vi "Do.vi"(8 "error in (no error)":errorcluster, 10 "Actor in":refnum<class "Actor.lvclass">, 11 "Set Delays Msg":refnum<class "Set Delays Msg.lvclass">) -> (0 "error out":errorcluster, 2 "Actor out":refnum<class "Actor.lvclass">)   [LabVIEW 2021, in "BNT_DAQmx.lvlib" / "Set Delays Msg.lvclass"]
doc: "This VI delivers the message to the actor by calling the appropriate method(s) on the actor."
uses:
  Set Delays Msg.lvclass
  <vilib>/ActorFramework/Actor/Actor.lvclass
  C:/Users/Holger/Documents/LVP/BNT/EQCR/Packages/CSPP_Core/Messages/CSPP_PVUpdate Msg/CSPP_PVUpdate Msg.lvclass
  BNT_DAQmx-MCSV-DOPWM/BNT_DAQmx-MCSV-DOPWM.lvclass
  C:/Program Files (x86)/National Instruments/LabVIEW 2021/vi.lib/ActorFramework/Actor/Actor.lvclass
  CSPP_Core/Messages/CSPP_PVUpdate Msg/CSPP_PVUpdate Msg.lvclass/CSPP_PVUpdate Msg.ctl
  CSPP_Core/Classes/CSPP_ProcessVariables/ProcessVariable/PV.lvclass/PV.ctl
  Set Delays Msg.lvclass/Set Delays Msg.ctl
  CSPP_Core/Classes/CSPP_ProcessVariables/ProcessVariable/PV.lvclass
  CSPP_Core/Messages/CSPP_PVUpdate Msg/CSPP_PVUpdate Msg.lvclass
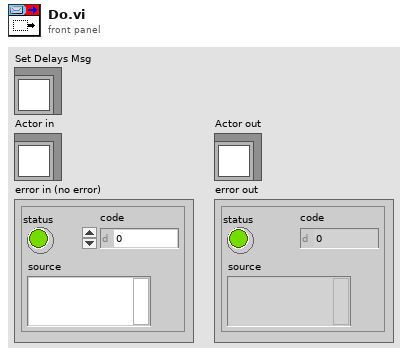
[diagram p1: front panel]
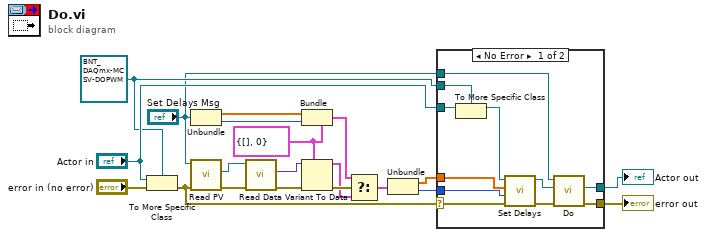
[diagram p0: block diagram]
diagram:
  w13 = cluster{"PWM Delays":dbl[], "Start Index":i32} {"PWM Delays"=[], "Start Index"=0} ("Type")
  w16 = refnum<class "BNT_DAQmx-MCSV-DOPWM.lvclass"> refnum ("Actor in")
  n1 = To More Specific Class(target class=w16, reference="Actor in", error in="error in (no error)") -> (error out=w10:errorcluster)  [unwired: 1 out]
  n2 = Unbundle ("Pre-Unbundler")("Set Delays Msg") -> (w2:dbl[], w1:i32)
  n3 = call "Read PV.vi"("error in (no error)"=w10, "CS++PVUpdate Msg in"="Set Delays Msg") -> ("error out"=w15:errorcluster, "PV"=w12:refnum<class "PV.lvclass">)  [unwired: 7 in, 1 out]
  n4 = call "Read Data.vi"("error in (no error)"=w15, "PV in"=w12) -> ("error out"=w6:errorcluster, "Data"=w5:variant)  [unwired: 7 in, 1 out]
  n5 = Bundle ("Pre-Bundler")(cluster=w13, "PWM Delays"=w2, "Start Index"=w1) -> (w7:cluster{"PWM Delays":dbl[], "Start Index":i32})
  n6 = Variant To Data(error in=w6, type=w13, Variant=w5) -> (data=w8:cluster{"PWM Delays":dbl[], "Start Index":i32}, error out=w14:errorcluster)
  n7 = Select ("MainSelect")(t=w7, s=w14, f=w8) -> (s? t:f=w11:cluster{"PWM Delays":dbl[], "Start Index":i32})
  n8 = Unbundle ("Main-Unbundler")(w11) -> ("PWM Delays"=w4:dbl[], "Start Index"=w3:i32)
  n9 = case shown="No Error" w10 {
    selector: w10 -> [w31 w33]
    tunnel: [w26 w33] -> w19
    tunnel: [w27 w32] -> w18
    tunnel: "Actor in" -> [w30 w32]
    tunnel: w16 -> [w29 _]
    tunnel: "Set Delays Msg" -> [w23 _]
    tunnel: w4 -> [w22 _]
    tunnel: w3 -> [w21 _]
    frame No Error {
      n10 = To More Specific Class ("To More Specific Class (internal)")(target class=w29, reference=w30) -> (specific class reference=w28:refnum<class "BNT_DAQmx-MCSV-DOPWM.lvclass">)  [unwired: 1 in, 1 out]
      n11 = call "Set Delays.vi"("error in"=w31, "Start Index"=w21, "PWM Delays"=w22, "BNT_DAQmx-MCSV-DOPWM in"=w28) -> ("error out"=w25:errorcluster, "BNT_DAQmx-MCSV-DOPWM out"=w24:refnum<class "BNT_DAQmx-MCSV-DOPWM.lvclass">)  [unwired: 6 in]
      n12 = call-parent "Do.vi"("error in (no error)"=w25, "Actor in"=w24, "CS++PVUpdate Msg"=w23) -> ("error out"=w26:errorcluster, "Actor out"=w27:refnum<class "Actor.lvclass">)  [unwired: 7 in]
    }
    frame Error {
    }
  }
  "error out" <- w19
  "Actor out" <- w18
